vi "postMSG.vi"(7 "station":string, 8 "error in (no error)":errorcluster caption="错误输入（无错误）", 9 "data":string[](array[string]), 10 "columns":string[](array[string]), 11 "table":string) -> (0 "error out":errorcluster caption="错误输出")   [LabVIEW 2016]
uses:
  <vilib>/httpClient/POSTBuffer.vi
  <vilib>/httpClient/LabVIEWHTTPClient.lvlib
panel:
  in  "debug":bool
  out "headers":string caption="头部"
  out "body":string caption="体部"
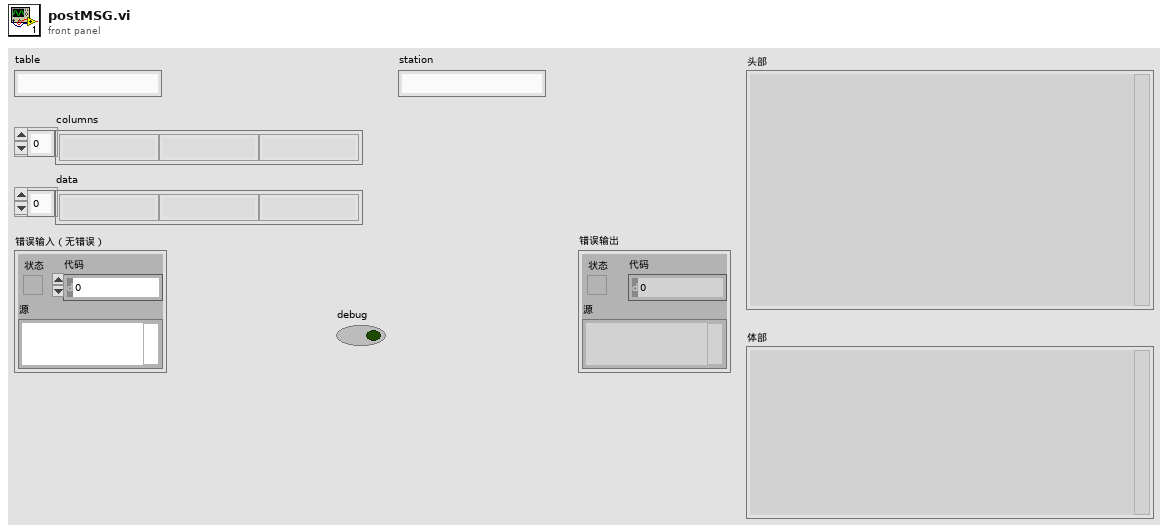
[diagram p1: front panel]
types:
  T1 = cluster{"station":string, "table":string, "columns":string[], "data":string[]}
  T2 = typedef "LabVIEWHTTPClient.lvlib/ClientHandle.ctl" = refnum<k1>
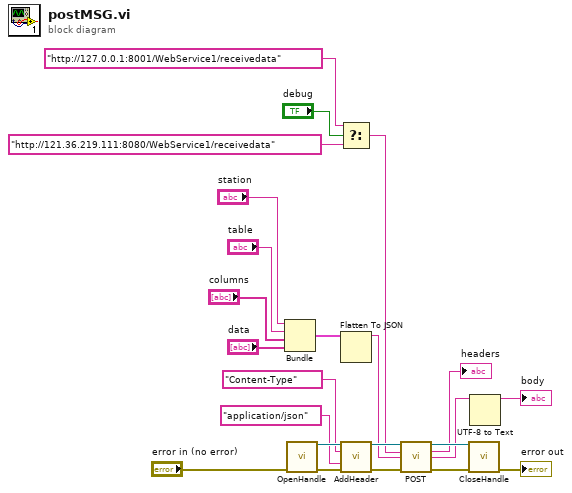
[diagram p0: block diagram]
diagram:
  n1 = Bundle("station"="station", "table"="table", "columns"="columns", "data"="data") -> (w8:T1)  [unwired: 1 in]
  n2 = call <vilib>:"OpenHandle.vi"("error in (no error)"="error in (no error)") -> ("client handle out"=w23:T2, "error out"=w21:errorcluster)  [unwired: 13 in]
  n3 = Select(t="http://127.0.0.1:8001/WebService1/receivedata" ("url"), s="debug", f="http://121.36.219.111:8080/WebService1/receivedata" ("url")) -> (s? t:f=w2:string)
  n4 = Flatten To JSON(anything=w8) -> (JSON string=w7:string)  [unwired: 2 in, 1 out]
  n5 = call <vilib>:"AddHeader.vi"("client handle"=w23, "header"="Content-Type", "value"="application/json", "error in (no error)"=w21) -> ("client handle out"=w22:T2, "error out"=w18:errorcluster)  [unwired: 10 in]
  n6 = call-poly <vilib>:"POST.vi"("client handle"=w22, "url"=w2, "buffer"=w7, "error in (no error)"=w18) -> ("client handle out"=w16:T2, "headers"=→"headers":string, "body"=w12:string, "error out"=w17:errorcluster)  [unwired: 8 in]
  n7 = call <vilib>:"CloseHandle.vi"("client handle"=w16, "error in (no error)"=w17) -> ("error out"=→"error out":errorcluster)  [unwired: 13 in]
  n8 = UTF-8 to Text(11:w12) -> (3:→"body":string)  [unwired: 2 in, 1 out]
